vi "Date and Time Attributes.vi"(0 "Timestamp (current)":timestamp) -> (1 "Attribute Names":string[](array[string]), 2 "Attribute Values":variant[](array[variant]), 3 "Timestamp out":timestamp)   [LabVIEW 2017]
doc: "Generates standard date and time attributes for easy incorporation into dataset or group attributes."
panel:
  # "LVHDF5 Toolkit\nCopyright (c) 2005-2013 by Jason D. Sommerville\nCopyright (c) 2014 by UPVI, LLC.\n\nThis use and distribution of this file is governed by the terms found in \nLICENSE.txt distributed with this toolkit and installed at\n <user.lib>\\_lvhdf5\\LICENSE.txt"
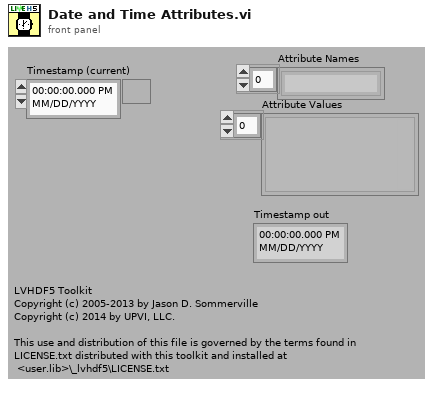
[diagram p1: front panel]
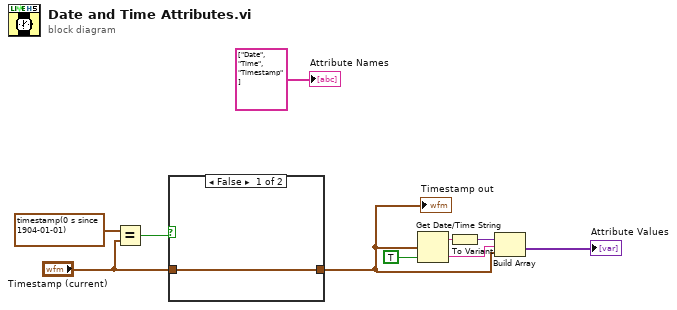
[diagram p0: block diagram]
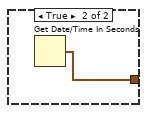
[diagram p2: hidden frame]
diagram:
  n1 = Equal?(x=timestamp(0 s since 1904-01-01) ("current time"), y="Timestamp (current)") -> (x = y?=w3:bool)
  n2 = case shown="False" w3 {
    tunnel: [w11 w12] -> w2
    tunnel: "Timestamp (current)" -> [w11 _]
    frame False {
    }
    frame True {
      n3 = Get Date/Time In Seconds() -> (seconds since 1Jan1904=w12:timestamp)
    }
  }
  "Timestamp out" <- w2
  n4 = Get Date/Time String(seconds (now)=w2, want seconds? (F)=TRUE) -> (date string=w6:string, time string=w7:string)  [unwired: 1 in]
  n5 = To Variant(anything=w6) -> (Variant=w10:variant)
  n6 = Build Array(w10, w7, w2) -> (→"Attribute Values":variant[])
  "Attribute Names" <- string[] ["Date", "Time", "Timestamp"]
